vi "Configuration Convert 1.0 to 1.1.vi"(8 "error in (no error)":errorcluster, 11 "framework configuration 1.0":T1) -> (0 "error out":errorcluster, 3 "framework configuration 1.1":T2={"Plugins"=[{"name"="Plugin", "components"=[], "cycle timing"={"priority"=10000, "decimation"=1, "offset"=0}, "threads"=[], "Transfer Groups"=[{"name"="Group", "direction"=enum."Tx", "cycle timing"={"priority"=100, "decimation"=1, "offset"=0}, "thread index"=-1, "settings"=[], "Transfers"=[{"name"="Transfer", "byte order"=enum."big-endian", "settings"=[], "channels"=[{"string offset"=0, "string data type"=enum."DBL", "engine data type"=enum."DBL", "name"="Channel", "settings"=[], "units"="V"}]}], "timeout behavior"=enum."Increment Late Count"}], "settings"=[]}]})   [LabVIEW 2017, in "DSF Core.lvlib" / "Configuration Session.lvclass"]
uses:
  Configuration Session.lvclass
  Configuration 1.1.ctl
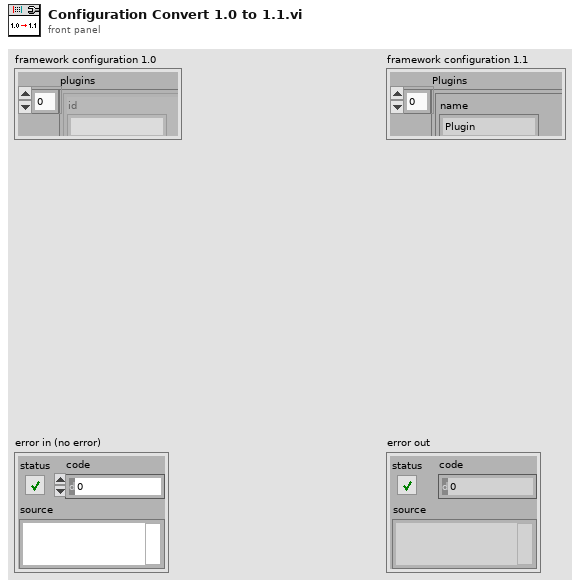
[diagram p1: front panel]
types:
  T1 = cluster{"plugins":cluster{"id":string, "values":cluster{"components":string[], "timing":cluster{"priority":u64, "decimation":u64, "offset":u64}, "group ids":string[], "settings id":string, "threads":cluster{"buffer converter settings":cluster{"key":string, "value":string}[], "transceiver settings":cluster{"key":string, "value":string}[], "custom settings":cluster{"key":string, "value":string}[], "processor":i32, "priority offset":i16}[]}}[], "groups":cluster{"id":string, "values":cluster{"direction":i32, "timing":cluster{"priority":u64, "decimation":u64, "offset":u64}, "transfer ids":string[], "settings id":string, "thread":i32, "timeout behavior":u8}}[], "transfers":cluster{"id":string, "values":cluster{"byte order":i32, "channel ids":string[], "settings id":string}}[], "channels":cluster{"id":string, "values":cluster{"string buffer offset":u64, "string data type":i32, "engine data type":i32, "settings id":string, "units":string}}[], "settings":cluster{"id":string, "values":cluster{"key":string, "value":string}[]}[]}
  T2 = typedef "DSF Core.lvlib/Configuration Session.lvclass/Configuration 1.1.ctl" = cluster{"Plugins":cluster{"name":string, "components":string[], "cycle timing":cluster{"priority":u64, "decimation":u64, "offset":u64}, "threads":cluster{"buffer converter settings":cluster{"key":string, "value":string}[], "transceiver settings":cluster{"key":string, "value":string}[], "custom settings":cluster{"key":string, "value":string}[], "processor":i32, "priority offset":i16}[], "Transfer Groups":cluster{"name":string, "direction":enum8{"Tx", "Rx"}, "cycle timing":cluster{"priority":u64, "decimation":u64, "offset":u64}, "thread index":i32, "settings":cluster{"key":string, "value":string}[], "Transfers":cluster{"name":string, "byte order":enum8{"big-endian", "little-endian"}, "settings":cluster{"key":string, "value":string}[], "channels":cluster{"string offset":u64, "string data type":enum8{"Bool", "SGL", "DBL", "I8", "I16", "I32", "I64", "U8", "U16", "U32", "U64"}, "engine data type":enum8{"Bool", "SGL", "DBL", "I8", "I16", "I32", "I64", "U8", "U16", "U32", "U64"}, "name":string, "settings":cluster{"key":string, "value":string}[], "units":string}[]}[], "timeout behavior":enum8{"Increment Late Count", "Throw Error"}}[], "settings":cluster{"key":string, "value":string}[]}[]}
  T3 = cluster{"name":string, "components":string[], "cycle timing":cluster{"priority":u64, "decimation":u64, "offset":u64}, "threads":cluster{"buffer converter settings":cluster{"key":string, "value":string}[], "transceiver settings":cluster{"key":string, "value":string}[], "custom settings":cluster{"key":string, "value":string}[], "processor":i32, "priority offset":i16}[], "Transfer Groups":cluster{"name":string, "direction":enum8{"Tx", "Rx"}, "cycle timing":cluster{"priority":u64, "decimation":u64, "offset":u64}, "thread index":i32, "settings":cluster{"key":string, "value":string}[], "Transfers":cluster{"name":string, "byte order":enum8{"big-endian", "little-endian"}, "settings":cluster{"key":string, "value":string}[], "channels":cluster{"string offset":u64, "string data type":enum8{"Bool", "SGL", "DBL", "I8", "I16", "I32", "I64", "U8", "U16", "U32", "U64"}, "engine data type":enum8{"Bool", "SGL", "DBL", "I8", "I16", "I32", "I64", "U8", "U16", "U32", "U64"}, "name":string, "settings":cluster{"key":string, "value":string}[], "units":string}[]}[], "timeout behavior":enum8{"Increment Late Count", "Throw Error"}}[], "settings":cluster{"key":string, "value":string}[]}
  T4 = cluster{"name":string, "direction":enum8{"Tx", "Rx"}, "cycle timing":cluster{"priority":u64, "decimation":u64, "offset":u64}, "thread index":i32, "settings":cluster{"key":string, "value":string}[], "Transfers":cluster{"name":string, "byte order":enum8{"big-endian", "little-endian"}, "settings":cluster{"key":string, "value":string}[], "channels":cluster{"string offset":u64, "string data type":enum8{"Bool", "SGL", "DBL", "I8", "I16", "I32", "I64", "U8", "U16", "U32", "U64"}, "engine data type":enum8{"Bool", "SGL", "DBL", "I8", "I16", "I32", "I64", "U8", "U16", "U32", "U64"}, "name":string, "settings":cluster{"key":string, "value":string}[], "units":string}[]}[], "timeout behavior":enum8{"Increment Late Count", "Throw Error"}}
  T5 = cluster{"name":string, "byte order":enum8{"big-endian", "little-endian"}, "settings":cluster{"key":string, "value":string}[], "channels":cluster{"string offset":u64, "string data type":enum8{"Bool", "SGL", "DBL", "I8", "I16", "I32", "I64", "U8", "U16", "U32", "U64"}, "engine data type":enum8{"Bool", "SGL", "DBL", "I8", "I16", "I32", "I64", "U8", "U16", "U32", "U64"}, "name":string, "settings":cluster{"key":string, "value":string}[], "units":string}[]}
  T6 = cluster{"string offset":u64, "string data type":enum8{"Bool", "SGL", "DBL", "I8", "I16", "I32", "I64", "U8", "U16", "U32", "U64"}, "engine data type":enum8{"Bool", "SGL", "DBL", "I8", "I16", "I32", "I64", "U8", "U16", "U32", "U64"}, "name":string, "settings":cluster{"key":string, "value":string}[], "units":string}
  T7 = cluster{"id":string, "values":cluster{"components":string[], "timing":cluster{"priority":u64, "decimation":u64, "offset":u64}, "group ids":string[], "settings id":string, "threads":cluster{"buffer converter settings":cluster{"key":string, "value":string}[], "transceiver settings":cluster{"key":string, "value":string}[], "custom settings":cluster{"key":string, "value":string}[], "processor":i32, "priority offset":i16}[]}}[]
  T8 = cluster{"id":string, "values":cluster{"direction":i32, "timing":cluster{"priority":u64, "decimation":u64, "offset":u64}, "transfer ids":string[], "settings id":string, "thread":i32, "timeout behavior":u8}}[]
  T9 = cluster{"id":string, "values":cluster{"byte order":i32, "channel ids":string[], "settings id":string}}[]
  T10 = cluster{"id":string, "values":cluster{"string buffer offset":u64, "string data type":i32, "engine data type":i32, "settings id":string, "units":string}}[]
  T11 = cluster{"id":string, "values":cluster{"key":string, "value":string}[]}[]
  T12 = cluster{"components":string[], "timing":cluster{"priority":u64, "decimation":u64, "offset":u64}, "group ids":string[], "settings id":string, "threads":cluster{"buffer converter settings":cluster{"key":string, "value":string}[], "transceiver settings":cluster{"key":string, "value":string}[], "custom settings":cluster{"key":string, "value":string}[], "processor":i32, "priority offset":i16}[]}
  T13 = cluster{"priority":u64, "decimation":u64, "offset":u64}
  T14 = cluster{"buffer converter settings":cluster{"key":string, "value":string}[], "transceiver settings":cluster{"key":string, "value":string}[], "custom settings":cluster{"key":string, "value":string}[], "processor":i32, "priority offset":i16}[]
  T15 = cluster{"direction":i32, "timing":cluster{"priority":u64, "decimation":u64, "offset":u64}, "transfer ids":string[], "settings id":string, "thread":i32, "timeout behavior":u8}
  T16 = cluster{"byte order":i32, "channel ids":string[], "settings id":string}
  T17 = cluster{"string buffer offset":u64, "string data type":i32, "engine data type":i32, "settings id":string, "units":string}
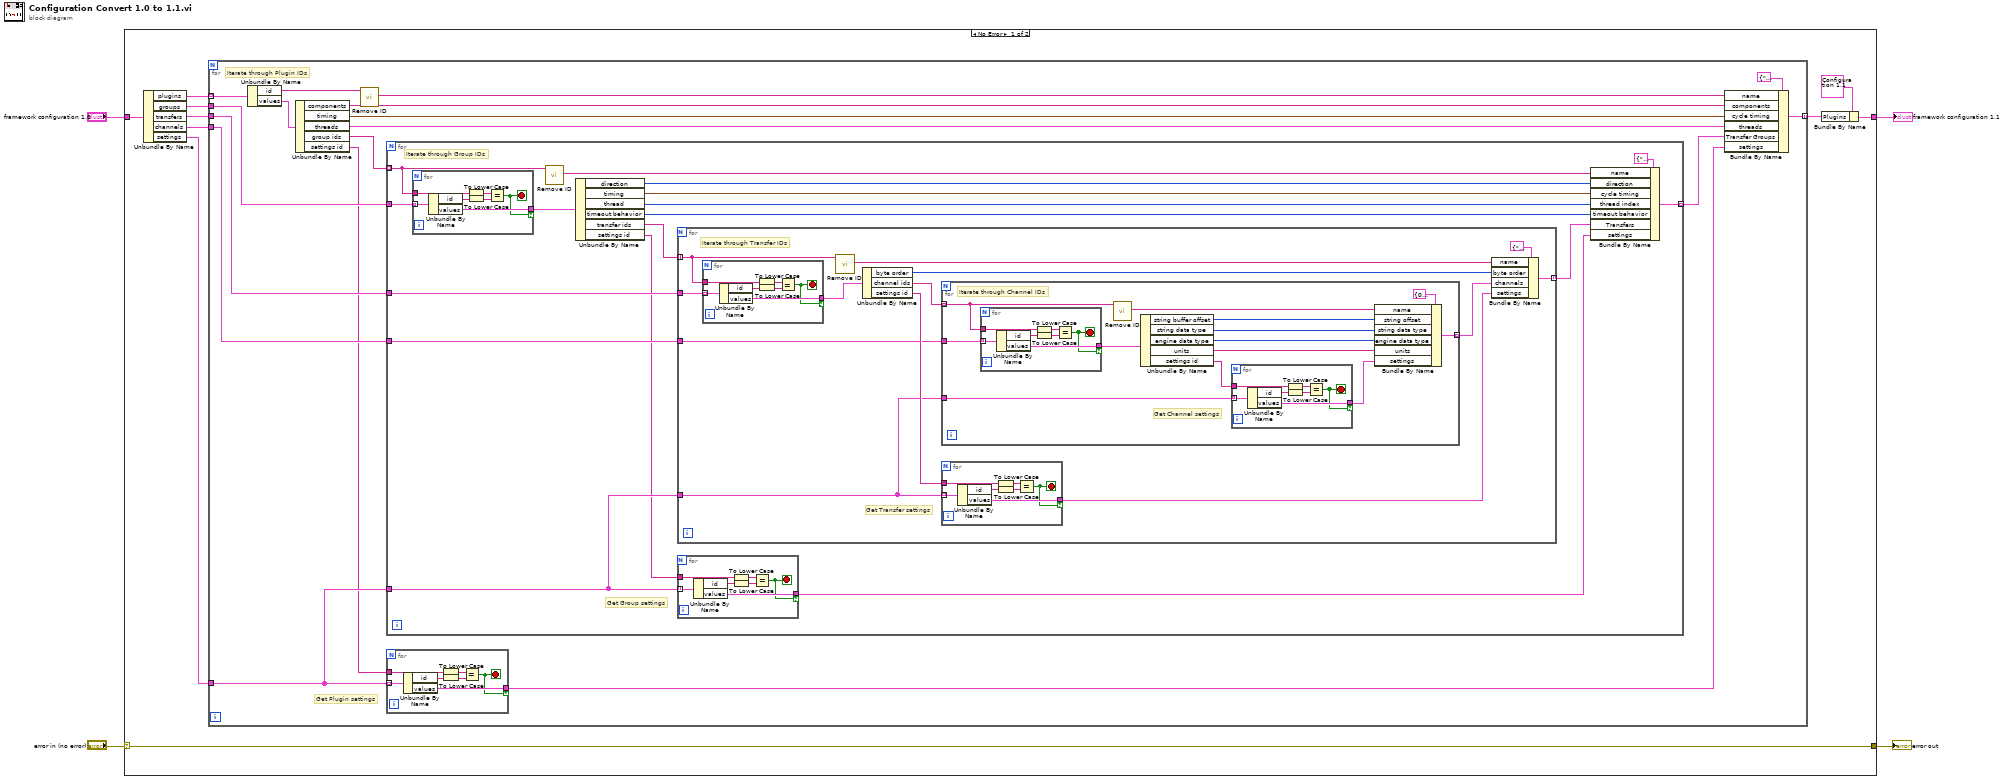
[diagram p0: block diagram]
diagram:
  n1 = case shown="No Error" "error in (no error)" {
    selector: "error in (no error)" -> [w5 w124]
    tunnel: [w5 w124] -> w4
    tunnel: "framework configuration 1.0" -> [w9 _]
    tunnel: [w7 _] -> w1
    frame No Error {
      n2 = Unbundle By Name(w9) -> ("plugins"=w13:T7, "groups"=w12:T8, "transfers"=w11:T9, "channels"=w10:T10, "settings"=w6:T11)
      n3 = for {
        tunnel: w13 -> [w31] mode=indexing
        tunnel: w12 -> [w19]
        tunnel: w11 -> [w18]
        tunnel: w10 -> [w17]
        tunnel: w6 -> [w16]
        tunnel: [w20] -> w8 mode=indexing
        # "Get Plugin settings"
        # "Iterate through Plugin IDs"
        n4 = Unbundle By Name(w31) -> ("id"=w28:string, "values"=w26:T12)
        n5 = Unbundle By Name(w26) -> ("components"=w25:string[], "timing"=w24:T13, "threads"=w23:T14, "group ids"=w22:string[], "settings id"=w15:string)
        n6 = call "Remove ID.vi"("id string"=w28) -> ("name"=w29:string)  [unwired: 8 in, 2 out]
        n7 = for {
          tunnel: w22 -> [w32] mode=indexing
          tunnel: w19 -> [w47]
          tunnel: w16 -> [w34]
          tunnel: [w39] -> w21 mode=indexing
          tunnel: w18 -> [w36]
          tunnel: w17 -> [w35]
          # "Get Group settings"
          # "Iterate through Group IDs"
          n8 = for {
            tunnel: w47 -> [w55] mode=indexing
            tunnel: [w52] -> w46 if=w49
            tunnel: w32 -> [w51]
            stop <- w49 stop-if-true
            n9 = Unbundle By Name(w55) -> ("id"=w53:string, "values"=w52:T15)
            n10 = To Lower Case(string=w51) -> (all lower case string=w50:string)
            n11 = To Lower Case(string=w53) -> (all lower case string=w54:string)
            n12 = Equal?(x=w50, y=w54) -> (x = y?=w49:bool)
          }
          n13 = call "Remove ID.vi"("id string"=w32) -> ("name"=w44:string)  [unwired: 8 in, 2 out]
          n14 = Unbundle By Name(w46) -> ("direction"=w45:i32, "timing"=w43:T13, "thread"=w42:i32, "timeout behavior"=w41:u8, "transfer ids"=w38:string[], "settings id"=w33:string)
          n15 = for {
            tunnel: w38 -> [w68] mode=indexing
            tunnel: [w65] -> w37 mode=indexing
            tunnel: w36 -> [w64]
            tunnel: w35 -> [w59]
            tunnel: w34 -> [w56]
            # "Get Transfer settings"
            # "Iterate through Transfer IDs"
            n16 = for {
              tunnel: w64 -> [w75] mode=indexing
              tunnel: [w72] -> w63 if=w69
              tunnel: w68 -> [w71]
              stop <- w69 stop-if-true
              n17 = Unbundle By Name(w75) -> ("id"=w73:string, "values"=w72:T16)
              n18 = To Lower Case(string=w71) -> (all lower case string=w70:string)
              n19 = To Lower Case(string=w73) -> (all lower case string=w74:string)
              n20 = Equal?(x=w70, y=w74) -> (x = y?=w69:bool)
            }
            n21 = call "Remove ID.vi"("id string"=w68) -> ("name"=w66:string)  [unwired: 8 in, 2 out]
            n22 = Unbundle By Name(w63) -> ("byte order"=w62:i32, "channel ids"=w60:string[], "settings id"=w61:string)
            n23 = for {
              tunnel: w60 -> [w87] mode=indexing
              tunnel: w59 -> [w85]
              tunnel: [w80] -> w57 mode=indexing
              tunnel: w56 -> [w79]
              # "Get Channel settings"
              # "Iterate through Channel IDs"
              n24 = for {
                tunnel: w85 -> [w95] mode=indexing
                tunnel: [w92] -> w84 if=w89
                tunnel: w87 -> [w91]
                stop <- w89 stop-if-true
                n25 = Unbundle By Name(w95) -> ("id"=w93:string, "values"=w92:T17)
                n26 = To Lower Case(string=w91) -> (all lower case string=w90:string)
                n27 = To Lower Case(string=w93) -> (all lower case string=w94:string)
                n28 = Equal?(x=w90, y=w94) -> (x = y?=w89:bool)
              }
              n29 = call "Remove ID.vi"("id string"=w87) -> ("name"=w86:string)  [unwired: 8 in, 2 out]
              n30 = Unbundle By Name(w84) -> ("string buffer offset"=w83:u64, "string data type"=w82:i32, "engine data type"=w76:i32, "units"=w81:string, "settings id"=w78:string)
              n31 = for {
                tunnel: w79 -> [w102] mode=indexing
                tunnel: [w99] -> w77 if=w97
                tunnel: w78 -> [w96]
                stop <- w97 stop-if-true
                n32 = Unbundle By Name(w102) -> ("id"=w100:string, "values"=w99:cluster{"key":string, "value":string}[])
                n33 = To Lower Case(string=w96) -> (all lower case string=w98:string)
                n34 = To Lower Case(string=w100) -> (all lower case string=w101:string)
                n35 = Equal?(x=w98, y=w101) -> (x = y?=w97:bool)
              }
              n36 = Bundle By Name(cluster=T6 {"string offset"=0, "string data type"=enum."Bool", "engine data type"=enum."Bool", "name"="", "settings"=[], "units"=""} ("channels"), "name"=w86, "string offset"=w83, "string data type"=w82, "engine data type"=w76, "units"=w81, "settings"=w77) -> (w80:T6)
            }
            n37 = for {
              tunnel: w56 -> [w109] mode=indexing
              tunnel: [w106] -> w58 if=w104
              tunnel: w61 -> [w103]
              stop <- w104 stop-if-true
              n38 = Unbundle By Name(w109) -> ("id"=w107:string, "values"=w106:cluster{"key":string, "value":string}[])
              n39 = To Lower Case(string=w103) -> (all lower case string=w105:string)
              n40 = To Lower Case(string=w107) -> (all lower case string=w108:string)
              n41 = Equal?(x=w105, y=w108) -> (x = y?=w104:bool)
            }
            n42 = Bundle By Name(cluster=T5 {"name"="", "byte order"=enum."big-endian", "settings"=[], "channels"=[]} ("Transfers"), "name"=w66, "byte order"=w62, "channels"=w57, "settings"=w58) -> (w65:T5)
          }
          n43 = for {
            tunnel: w34 -> [w116] mode=indexing
            tunnel: [w113] -> w40 if=w110
            tunnel: w33 -> [w112]
            stop <- w110 stop-if-true
            n44 = Unbundle By Name(w116) -> ("id"=w114:string, "values"=w113:cluster{"key":string, "value":string}[])
            n45 = To Lower Case(string=w112) -> (all lower case string=w111:string)
            n46 = To Lower Case(string=w114) -> (all lower case string=w115:string)
            n47 = Equal?(x=w111, y=w115) -> (x = y?=w110:bool)
          }
          n48 = Bundle By Name(cluster=T4 {"name"="", "direction"=enum."Tx", "cycle timing"={"priority"=0, "decimation"=0, "offset"=0}, "thread index"=0, "settings"=[], "Transfers"=[], "timeout behavior"=enum."Increment Late Count"} ("Transfer Groups"), "name"=w44, "direction"=w45, "cycle timing"=w43, "thread index"=w42, "timeout behavior"=w41, "Transfers"=w37, "settings"=w40) -> (w39:T4)
        }
        n49 = for {
          tunnel: w16 -> [w123] mode=indexing
          tunnel: [w120] -> w27 if=w117
          tunnel: w15 -> [w119]
          stop <- w117 stop-if-true
          n50 = Unbundle By Name(w123) -> ("id"=w121:string, "values"=w120:cluster{"key":string, "value":string}[])
          n51 = To Lower Case(string=w119) -> (all lower case string=w118:string)
          n52 = To Lower Case(string=w121) -> (all lower case string=w122:string)
          n53 = Equal?(x=w118, y=w122) -> (x = y?=w117:bool)
        }
        n54 = Bundle By Name(cluster=T3 {"name"="", "components"=[], "cycle timing"={"priority"=0, "decimation"=0, "offset"=0}, "threads"=[], "Transfer Groups"=[], "settings"=[]} ("Plugin Configuration"), "name"=w29, "components"=w25, "cycle timing"=w24, "threads"=w23, "Transfer Groups"=w21, "settings"=w27) -> (w20:T3)
      }
      n55 = Bundle By Name(cluster=T2 {"Plugins"=[{"name"="Plugin", "components"=[], "cycle timing"={"priority"=10000, "decimation"=1, "offset"=0}, "threads"=[], "Transfer Groups"=[{"name"="Group", "direction"=enum."Tx", "cycle timing"={"priority"=100, "decimation"=1, "offset"=0}, "thread index"=-1, "settings"=[], "Transfers"=[{"name"="Transfer", "byte order"=enum."big-endian", "settings"=[], "channels"=[{"string offset"=0, "string data type"=enum."DBL", "engine data type"=enum."DBL", "name"="Channel", "settings"=[], "units"="V"}]}], "timeout behavior"=enum."Increment Late Count"}], "settings"=[]}]} ("framework configuration 1.1"), "Plugins"=w8) -> (w7:T2)
    }
    frame Error {
    }
  }
  "error out" <- w4
  "framework configuration 1.1" <- w1
